vi "ActionVIOnCompile.vi"(8 "error in (no error)":errorcluster, 11 "Device Item Ref in":T1 format="%.0x") -> (0 "error out":errorcluster)   [LabVIEW 2026, in "WebPage Addon System Explorer.lvlib"]
uses:
  WebPage Addon System Explorer.lvlib
  <vilib>/NI VeriStand/Custom Device API/Custom Device Item Ref.ctl
  Addon Shared/Types/Compiled.Settings.ctl
  Types/Page Settings Action.ctl
  <vilib>/NI VeriStand/Custom Device API/Set Item Property (Variant).vi
  <vilib>/NI VeriStand/Custom Device API/Custom Device API.lvlib
  <vilib>/NI/NIVS Inline Async API/_Data Access System Explorer/Data Access System Explorer.lvlib
  Addon Shared/WebPage Addon Shared.lvlib
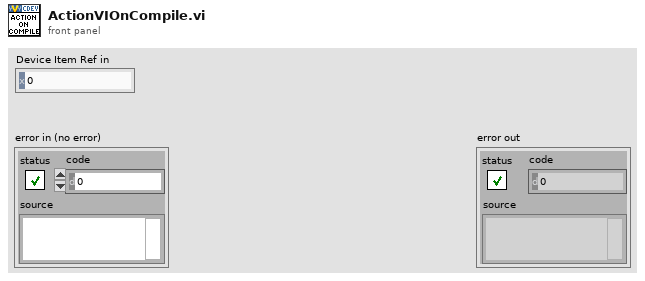
[diagram p1: front panel]
types:
  T1 = typedef "Custom Device API.lvlib/Custom Device Item Ref.ctl" = u64
  T2 = typedef "WebPage Addon System Explorer.lvlib/Page Settings Action.ctl" = enum16{"Get", "Set"}
  T3 = enum16{"Output/Write", "Input/Read", "Input/ReadWrite"}
  T4 = cluster{"Name":string, "Type":enum16{"Output/Write", "Input/Read", "Input/ReadWrite"}, "VS Refs":T1[]}
  T5 = typedef "WebPage Addon Shared.lvlib/Compiled.Settings.ctl" = cluster{"Name":string, "Decimation":u32, "Channel Names":string[], "Hosted IP Address":string, "Hosted Port":u32, "gRPC Port":u32}
  T6 = typedef "Custom Device API.lvlib/Custom Device Item Info.ctl" = cluster{"Name":string, "Is Channel":bool, "GUID":string, "Is Waveform":bool}
  T7 = typedef "WebPage Addon System Explorer.lvlib/Main.Settings.ctl" = cluster{"Update Rate":dbl, "Hosted Port":u32, "gRPC Port":u32, "Hosted IP Address":string}
  T8 = cluster{"Name":string, "Type":enum16{"Output/Write", "Input/Read", "Input/ReadWrite"}, "VS Refs":T1[]}[]
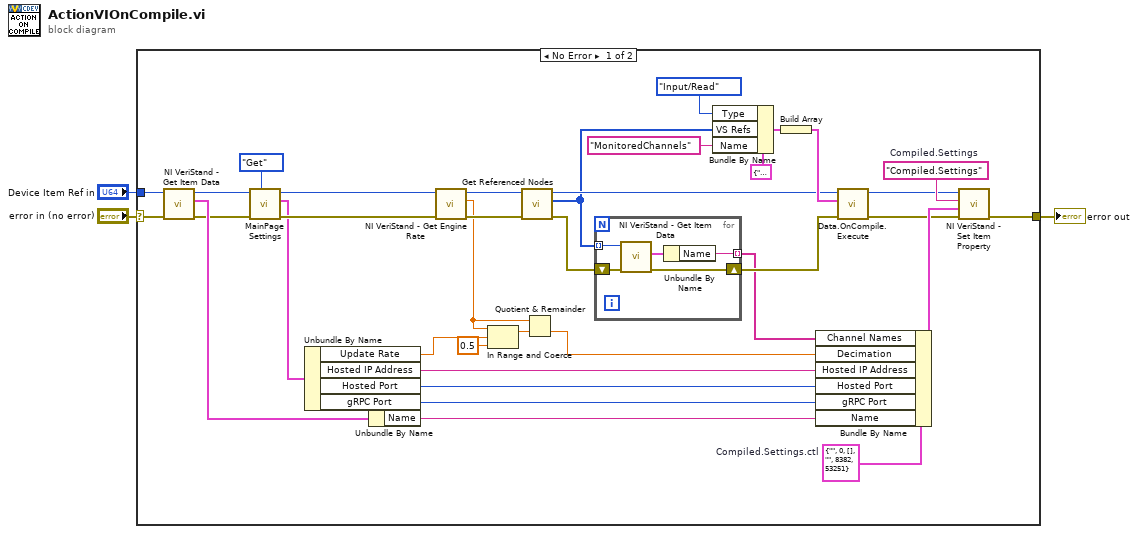
[diagram p0: block diagram]
diagram:
  n1 = case shown="No Error" "error in (no error)" {
    selector: "error in (no error)" -> [w36 w45]
    tunnel: [w37 w45] -> w2
    tunnel: "Device Item Ref in" -> [w35 _]
    frame No Error {
      w25 = T5 {"Name"="", "Decimation"=0, "Channel Names"=[], "Hosted IP Address"="", "Hosted Port"=8382, "gRPC Port"=53251}  # Compiled.Settings.ctl
      w39 = "Compiled.Settings"  # Compiled.Settings
      n2 = call <vilib>:"NI VeriStand - Get Item Data.vi"("error in (no error)"=w36, "Item Ref in"=w35) -> ("error out"=w12:errorcluster, "Item Info"=w34:T6, "Item Ref out"=w13:T1)  [unwired: 6 in, 1 out]
      n3 = call "MainPage Settings.vi"("Action"=Page_Settings_Action."Get", "error in (no error)"=w12, "Item Ref in"=w13) -> ("error out"=w10:errorcluster, "Settings Out"=w8:T7, "Item Ref out"=w9:T1)  [unwired: 6 in]
      n4 = Unbundle By Name(w8) -> ("Update Rate"=w7:dbl, "Hosted IP Address"=w6:string, "Hosted Port"=w5:u32, "gRPC Port"=w4:u32)
      n5 = Unbundle By Name(w34) -> ("Name"=w33:string)
      n6 = call <vilib>:"NI VeriStand - Get Engine Rate.vi"("error in (no error)"=w10, "Item Ref in"=w9) -> ("error out"=w23:errorcluster, "Rate (Hz)"=w20:dbl, "Item Ref out"=w22:T1)  [unwired: 7 in]
      n7 = In Range and Coerce(upper limit=w20, x=w7, lower limit=0.5) -> (coerced(x)=w19:dbl)  [unwired: 1 out]
      n8 = call "Get Referenced Nodes.vi"("error in (no error)"=w23, "Item Ref in"=w22) -> ("error out"=w17:errorcluster, "Array"=w15:T1[], "Item Ref out"=w24:T1)  [unwired: 7 in]
      n9 = Quotient & Remainder(x=w20, y=w19) -> (floor(x/y)=w18:dbl)  [unwired: 1 out]
      n10 = for {
        shift-right: [w43] -> w16
        shift-left: w17 -> [w44]
        tunnel: w15 -> [w42] mode=indexing
        tunnel: [w40] -> w14 mode=indexing
        n11 = call <vilib>:"NI VeriStand - Get Item Data.vi"("error in (no error)"=w44, "Item Ref in"=w42) -> ("error out"=w43:errorcluster, "Item Info"=w41:T6)  [unwired: 6 in, 2 out]
        n12 = Unbundle By Name(w41) -> ("Name"=w40:string)
      }
      n13 = Bundle By Name(cluster=T4 {"Name"="", "Type"=enum."Output/Write", "VS Refs"=[]} ("Group"), "Type"=T3."Input/Read", "VS Refs"=w15, "Name"="MonitoredChannels" ("Item Name")) -> (w28:T4)
      n14 = Build Array(w28) -> (w30:T8)
      n15 = Bundle By Name(cluster=w25, "Channel Names"=w14, "Decimation"=w18, "Hosted IP Address"=w6, "Hosted Port"=w5, "gRPC Port"=w4, "Name"=w33) -> (w38:T5)
      n16 = call <vilib>:"Data.OnCompile.Execute.vi"("error in"=w16, "VS Ref Groups"=w30, "Custom Device Ref"=w24) -> ("error out"=w27:errorcluster, "Custom Device Ref"=w26:T1)  [unwired: 7 in]
      n17 = call-poly <vilib>:"NI VeriStand - Set Item Property.vi"("error in (no error)"=w27, "Value"=w38, "Property Name"=w39, "Item Ref in"=w26) -> ("error out"=w37:errorcluster)  [unwired: 5 in, 2 out]
    }
    frame Error {
    }
  }
  "error out" <- w2
